vi "monitor poc.vi"(8 "error in":errorcluster, 9 "Active Channel":string, 10 "power monitor queue in":refnum<queue>, 11 "fpga interface in":refnum<k20>) -> (0 "error out":errorcluster)   [LabVIEW 2025, in "Automotive Vision.lvclass"]
uses:
  power.ctl
  <instrlib>/FlexRIO/API/Host/v1/NI FlexRIO/API/Get Property Reference - Fpga Small.vi
  Automotive Vision.lvclass
  Automotive Vision.lvclass/Automotive Vision.ctl
  <resource>/objmgr/niflexrioapiChannel.rc
  <instrlib>/FlexRIO/API/Host/v1/NI FlexRIO API v1.lvlib
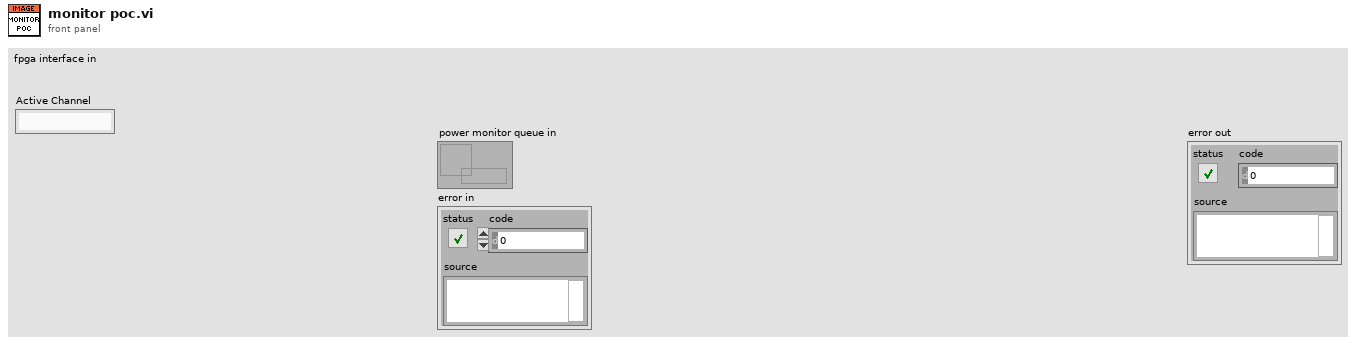
[diagram p1: front panel]
types:
  T1 = typedef "Automotive Vision.lvclass/power.ctl" = cluster{"Voltage":dbl, "Current":dbl}
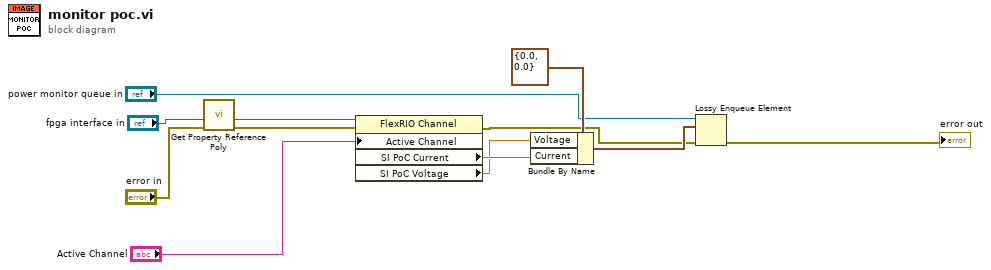
[diagram p0: block diagram]
diagram:
  n1 = call-poly <instrlib>:"Get Property Reference Poly.vi"("error in (no error)"="error in", "fpga interface in"="fpga interface in") -> ("error out"=w10:errorcluster, "property reference"=w11:refnum<k20>)  [unwired: 4 in, 1 out]
  n2 = property on="Property Node" class="FlexRIO Channel"(reference=w11, error in=w10, "Active Channel"="Active Channel") -> (error out=w3:errorcluster, "SI PoC Current"=w7:dbl, "SI PoC Voltage"=w6:dbl)  [unwired: 1 out]
  n3 = Bundle By Name(cluster=T1 {"Voltage"=0.0, "Current"=0.0} ("Power"), "Voltage"=w6, "Current"=w7) -> (w4:T1)
  n4 = Lossy Enqueue Element(queue="power monitor queue in", element=w4, error in (no error)=w3) -> (error out=→"error out":errorcluster)  [unwired: 3 out]
